vi "Teleop.vi"(10 "Match Info":T1={"Autonomous Elapsed Seconds"=0.0, "TeleOp Elapsed Seconds"=0.0, "Disabled Elapsed Seconds"=0.0, "Visited Autonomous"=FALSE, "Visited TeleOp"=FALSE, "Visited Disabled"=FALSE, "Autonomous Settings"={"Autonomous Style"=enum."Independent", "VI Refnum"=refnum}}) -> ()   [LabVIEW 2016]
doc: "This VI is called for each TeleOp packet received from the DS where the robot is not disabled. It is often used to read from the joysticks and update I/O or to update setpoints for timed control loops. It should complete and return within 20 milliseconds or it may miss DS packets."
uses:
  <vilib>/Rock Robotics/WPI/DriverStation/WPI_DriverStationMatch Info.ctl
  <vilib>/Rock Robotics/WPI/Utilities/WPI_GetSetVariantRefNum.vi
  <vilib>/Rock Robotics/Network Tables/NT Write Boolean Array.vi
  <vilib>/Rock Robotics/Network Tables/NT Write Numeric Array.vi
  <vilib>/Rock Robotics/Network Tables/NT Read Boolean.vi
  <vilib>/Rock Robotics/Network Tables/NT Read Number.vi
  encoderdirection1.vi
  encoder1.vi
panel:
  in  "Maximum":dbl
  in  "Minimum":dbl
  out "Boolean":bool
  in  "Numeric 2":dbl=0.5
  out "Sample Slider 0":dbl(slide) scale=0.0..5.0
  out "Sample Boolean 1":bool
  out "Sample Boolean 0":bool
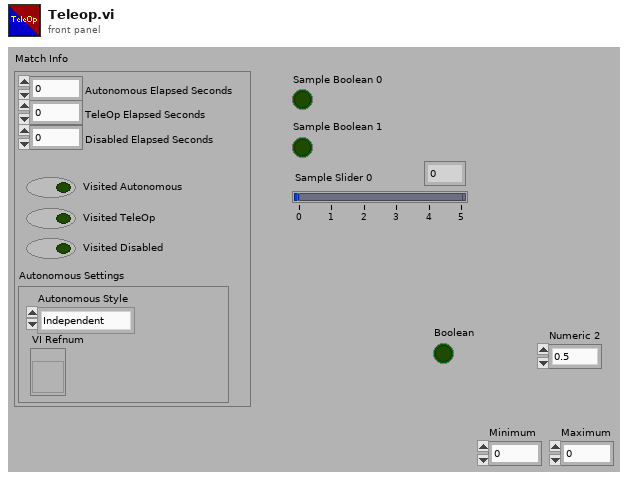
[diagram p1: front panel]
types:
  T1 = typedef "WPI_DriverStationMatch Info.ctl" = cluster{"Autonomous Elapsed Seconds":dbl, "TeleOp Elapsed Seconds":dbl, "Disabled Elapsed Seconds":dbl, "Visited Autonomous":bool, "Visited TeleOp":bool, "Visited Disabled":bool, "Autonomous Settings":cluster{"Autonomous Style":enum16{"Iterative", "Independent"}, "VI Refnum":refnum<vi>}}
  T2 = typedef "WPI_RobotDriveDevRef.ctl" = cluster{"DevStatus":errorcluster, "Motors[]":T3[], "Square Inputs":bool, "Max Output":dbl}
  T3 = typedef "WPI_MotorControlDeviceRef.ctl" = cluster{"DeviceStatus":errorcluster, "Type":T4, "PWM":cluster{"PWM Channel":T5, "DeadBand":T6}, "CAN":cluster{"Device Number":u8, "SetOutput VI Ref":variant, "GetOutput VI Ref":variant, "Enable VI Ref":variant, "Disable VI Ref":variant, "Data":variant}, "Invert":bool}
  T4 = typedef "WPI_MotorControlType.ctl" = enum16{"PWM", "CAN"}
  T5 = typedef "FPGA_DIOPWMChannel.ctl" = enum8{"PWM 0", "PWM 1", "PWM 2", "PWM 3", "PWM 4", "PWM 5", "PWM 6", "PWM 7", "PWM 8", "PWM 9", "PWM MXP 0", "PWM MXP 1", "PWM MXP 2", "PWM MXP 3", "PWM MXP 4", "PWM MXP 5", "PWM MXP 6", "PWM MXP 7", "PWM MXP 8", "PWM MXP 9", "Invalid"}
  T6 = typedef "WPI_PWMDeadband.ctl" = cluster{"Name":string, "maxPositivePwm":i32, "minPositivePwm":i32, "centerPwm":i32, "maxNegativePwm":i32, "minNegativePwm":i32, "angularRange":u16}
  T7 = typedef "WPI_JoystickDevRef.ctl" = cluster{"Device":T8}
  T8 = typedef "WPI_JoystickDeviceEnum.ctl" = enum16{"USB 0", "USB 1", "USB 2", "USB 3", "USB 4", "USB 5"}
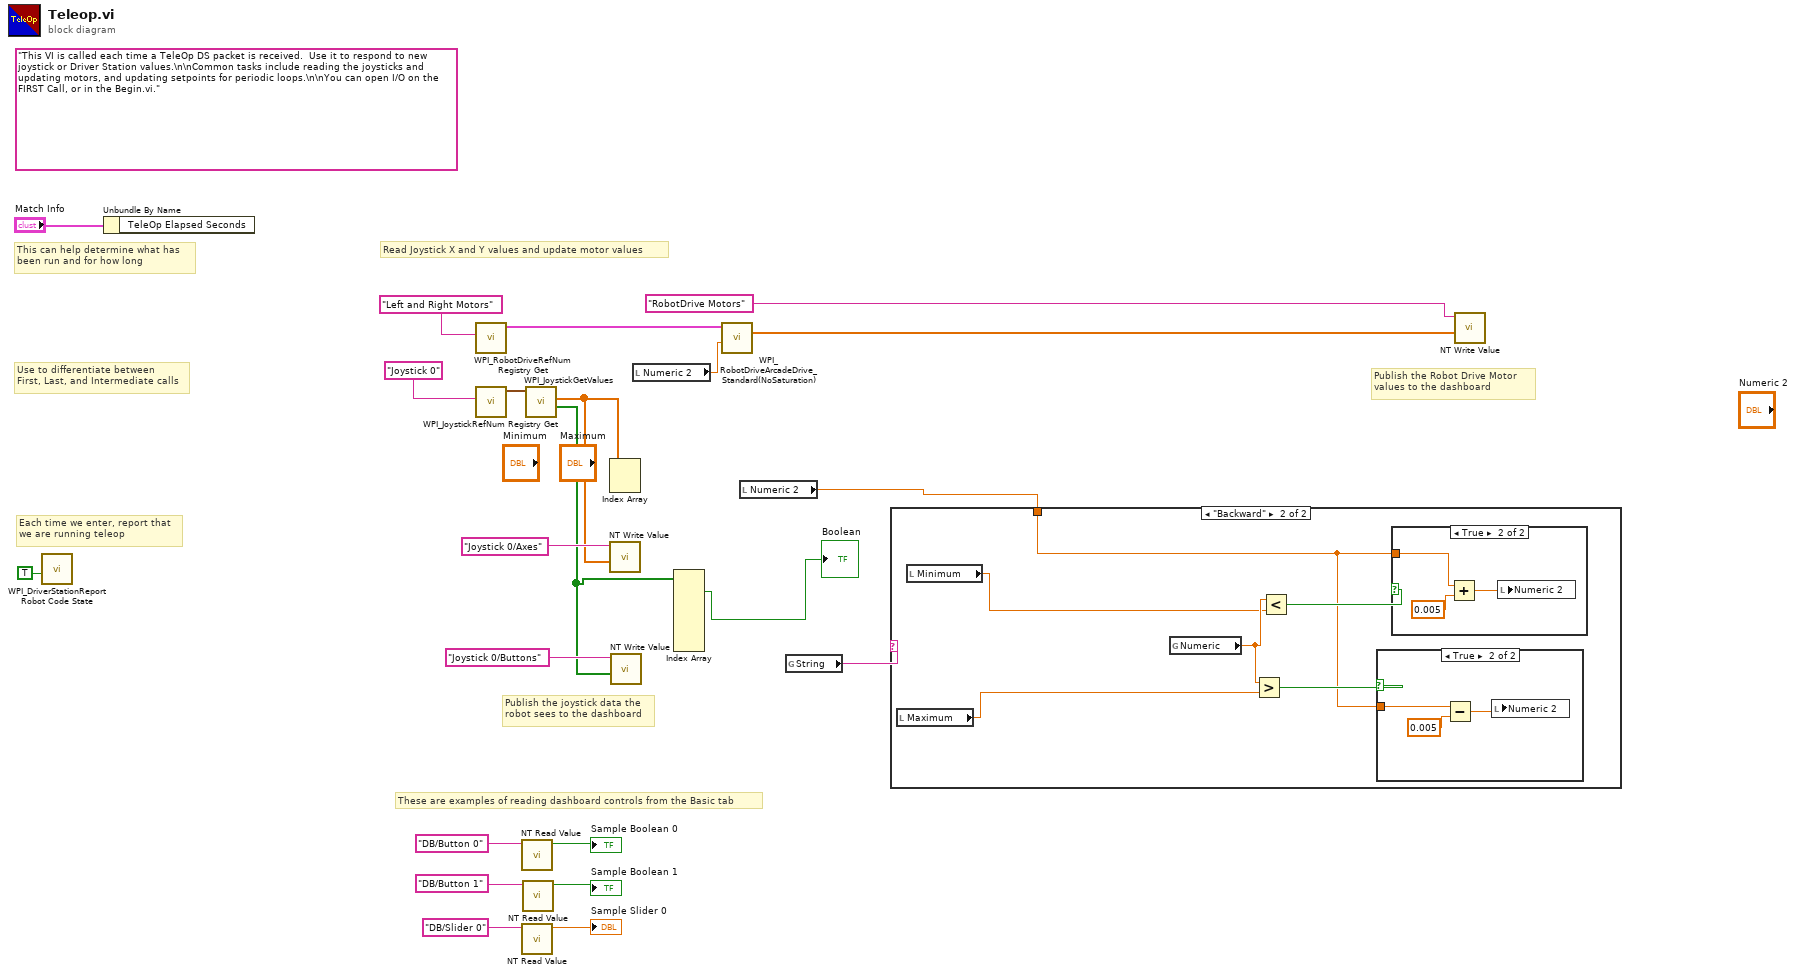
[diagram p0: block diagram]
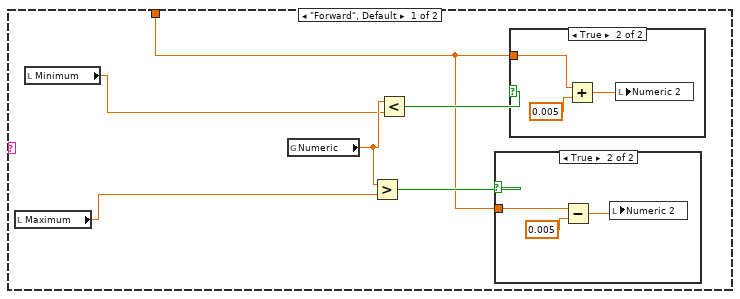
[diagram p2: hidden frame]
diagram:
  (unwired) "This VI is called each time a TeleOp DS packet is received.  Use it to respond to new joystick or Driver Station values.\n\nCommon tasks include reading the joysticks and updating motors, and updating setpoints for periodic loops.\n\nYou can open I/O on the FIRST Call, or in the Begin.vi."
  # "These are examples of reading dashboard controls from the Basic tab"
  # "Publish the Robot Drive Motor\nvalues to the dashboard"
  # "Publish the joystick data the\nrobot sees to the dashboard"
  # "Each time we enter, report that\nwe are running teleop"
  # "Use to differentiate between\nFirst, Last, and Intermediate calls"
  # "This can help determine what has\nbeen run and for how long"
  # "Read Joystick X and Y values and update motor values"
  n1 = call <vilib>:"WPI_DriverStationReport Robot Code State.vi"("TeleOp"=TRUE ("Autonomous")) -> ()  [unwired: 10 in, 1 out]
  n2 = Unbundle By Name("Match Info") -> ()  [unwired: 1 out]
  n3 = call <vilib>:"WPI_RobotDriveRefNum Registry Get.vi"("refnum name"="Left and Right Motors") -> ("RobotDriveDevRef"=w20:T2)  [unwired: 1 in, 9 out]
  n4 = call <vilib>:"WPI_JoystickRefNum Registry Get.vi"("refnum name"="Joystick 0") -> ("JoystickDevRef"=w18:T7)  [unwired: 1 in, 9 out]
  n5 = call-poly <vilib>:"NT Read Value.vi"("Name"="DB/Button 0" ("refnum name")) -> ("Boolean"=→"Sample Boolean 0":bool)  [unwired: 9 in, 1 out]
  n6 = call-poly <vilib>:"NT Read Value.vi"("Name"="DB/Slider 0" ("refnum name")) -> ("Numeric"=→"Sample Slider 0":dbl)  [unwired: 9 in, 1 out]
  n7 = call-poly <vilib>:"NT Read Value.vi"("Name"="DB/Button 1" ("refnum name")) -> ("Boolean"=→"Sample Boolean 1":bool)  [unwired: 9 in, 1 out]
  n8 = call <vilib>:"WPI_JoystickGetValues.vi"("JoystickDevRef"=w18) -> ("Buttons"=w5:bool[], "Axes"=w14:dbl[])  [unwired: 6 in, 3 out]
  n9 = Index Array(array=w14) -> ()  [unwired: 2 in, 2 out]
  n10 = call-poly <vilib>:"NT Write Value.vi"("Numeric Array"=w14, "Name"="Joystick 0/Axes") -> ()  [unwired: 9 in, 1 out]
  n11 = call-poly <vilib>:"NT Write Value.vi"("Boolean Array"=w5, "Name"="Joystick 0/Buttons") -> ()  [unwired: 9 in, 1 out]
  n12 = local read "Numeric 2"() -> (w1:dbl)
  n13 = Index Array(array=w5) -> (element #1=→"Boolean":bool)  [unwired: 8 in, 7 out]
  n14 = call <vilib>:"WPI_RobotDriveArcadeDrive_Standard(NoSaturation).vi"("Y axis value"=w1, "RobotDriveDevRef"=w20) -> ("Motor Values"=w7:dbl[])  [unwired: 2 in, 7 out]
  n15 = local read "Numeric 2"() -> (w3:dbl)
  n16 = global read "encoderdirection1.vi" "String"() -> (w2:string)
  n17 = case shown="\"Backward\"" w2 {
    tunnel: w3 -> [w25 w37]
    frame "Forward", Default {
      n18 = local read "Maximum"() -> (w23:dbl)
      n19 = local read "Minimum"() -> (w24:dbl)
      n20 = global read "encoder1.vi" "Numeric"() -> (w26:dbl)
      n21 = Greater?(x=w26, y=w23) -> (0:w27:bool)
      n22 = Less?(x=w26, y=w24) -> (x < y?=w28:bool)
      n23 = case shown="True" w27 {
        tunnel: w25 -> [_ w29]
        frame False {
        }
        frame True {
          n24 = Subtract(x=w29, y=0.005) -> (x-y=w30:dbl)
          n25 = local write "Numeric 2"(w30) -> ()
        }
      }
      n26 = case shown="True" w28 {
        tunnel: w25 -> [_ w32]
        frame False {
        }
        frame True {
          n27 = Add(x=w32, y=0.005) -> (x+y=w33:dbl)
          n28 = local write "Numeric 2"(w33) -> ()
        }
      }
    }
    frame "Backward" {
      n29 = local read "Maximum"() -> (w35:dbl)
      n30 = local read "Minimum"() -> (w36:dbl)
      n31 = global read "encoder1.vi" "Numeric"() -> (w38:dbl)
      n32 = Greater?(x=w38, y=w35) -> (0:w39:bool)
      n33 = Less?(x=w38, y=w36) -> (x < y?=w40:bool)
      n34 = case shown="True" w39 {
        tunnel: w37 -> [_ w41]
        frame False {
        }
        frame True {
          n35 = Subtract(x=w41, y=0.005) -> (x-y=w42:dbl)
          n36 = local write "Numeric 2"(w42) -> ()
        }
      }
      n37 = case shown="True" w40 {
        tunnel: w37 -> [_ w44]
        frame False {
        }
        frame True {
          n38 = Add(x=w44, y=0.005) -> (x+y=w45:dbl)
          n39 = local write "Numeric 2"(w45) -> ()
        }
      }
    }
  }
  n40 = call-poly <vilib>:"NT Write Value.vi"("Numeric Array"=w7, "Name"="RobotDrive Motors") -> ()  [unwired: 9 in, 1 out]
